vi "Read Key Values.vi"(8 "error in (no error)":errorcluster, 11 "Configuration in":refnum<class "Configuration.lvclass">) -> (0 "error out":errorcluster, 2 "Key Values":string[](array[string]), 3 "Configuration out":refnum<class "Configuration.lvclass">)   [LabVIEW 2023, in "Configuration.lvlib" / "Configuration.lvclass"]
doc: "Returns an array of key values - This is a placeholder for the configuration editor application."
uses:
  Library/Configuration.lvclass
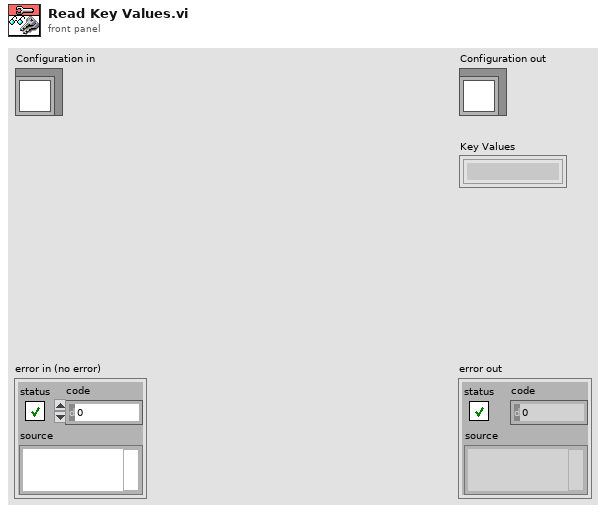
[diagram p1: front panel]
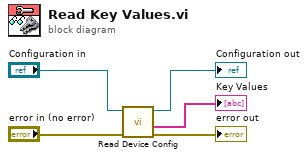
[diagram p0: block diagram]
diagram:
  n1 = call "Read Device Config.vi"("error in (no error)"="error in (no error)", "Configuration in"="Configuration in") -> ("error out"=→"error out":errorcluster, "Values"=→"Key Values":string[], "Configuration out"=→"Configuration out":refnum<class "Configuration.lvclass">)  [unwired: 6 in, 1 out]
